vi "read_settings_file.vi"(8 "error in (no error)":errorcluster, 9 "settings cluster in":variant, 10 "settings name":string, 11 "GenericPlugin in":refnum<class "ComponentTemplate.lvclass">) -> (0 "error out":errorcluster, 1 "settings cluster out":variant, 3 "GenericPlugin out":refnum<class "ComponentTemplate.lvclass">)   [LabVIEW 2010]
uses:
  ComponentTemplate.lvclass
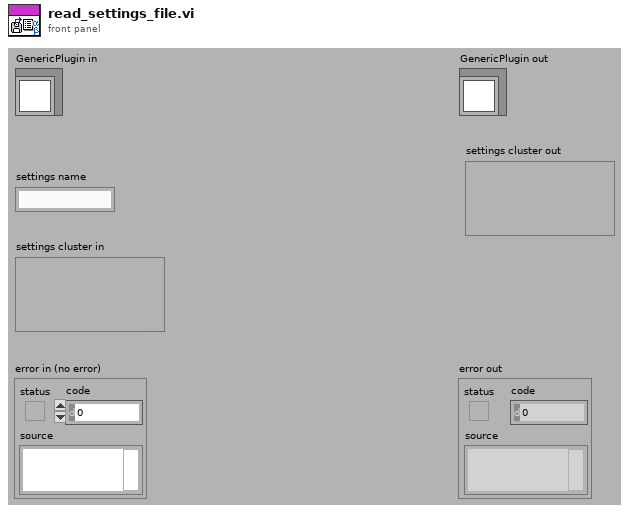
[diagram p1: front panel]
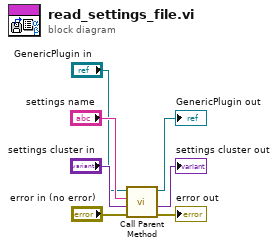
[diagram p0: block diagram]
diagram:
  n1 = call-parent "Call Parent Method"("error in (no error)"="error in (no error)", "settings cluster in"="settings cluster in", "settings name"="settings name", "GenericPlugin in"="GenericPlugin in") -> ("error out"=→"error out":errorcluster, "settings cluster out"=→"settings cluster out":variant, "GenericPlugin out"=→"GenericPlugin out":refnum<class "ComponentTemplate.lvclass">)  [unwired: 5 in]
